vi "Arrange Panels.vi"(8 "error in":errorcluster, 11 "cPAS Facade in":refnum<class "cPAS Facade.lvclass">) -> (0 "error out":errorcluster, 3 "cPAS Facade out":refnum<class "cPAS Facade.lvclass">)   [LabVIEW 2015, in "cPAS Facade.lvclass"]
uses:
  cPAS Facade.lvclass
  UIs.ctl
  Reusable/GUI/Facade/GUI Facade.lvclass/GUI Facade.ctl
  Reusable/GUI/Facade/Accessors/Read sPanel.vi
  Reusable/GUI/Facade/Accessors/Read FP Refs.vi
  Reusable/GUI/Facade/Accessors/Write sPanel.vi
  Reusable/GUI/Facade/Accessors/Write FP Refs.vi
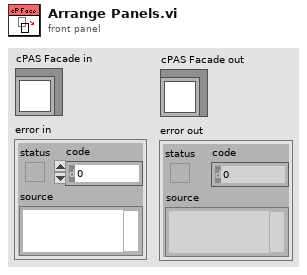
[diagram p1: front panel]
types:
  T1 = typedef "cPAS Facade.lvclass/UIs.ctl" = enum8{"PAS HF", "PAS Ctl", "PAS Der", "PAS HK", "Common", "Pcal", "CRD Ctl", "CRD RD", "CRD Der", "CRD HK", "Calibration", "CLAP", "Derived", "Housekeeping"}
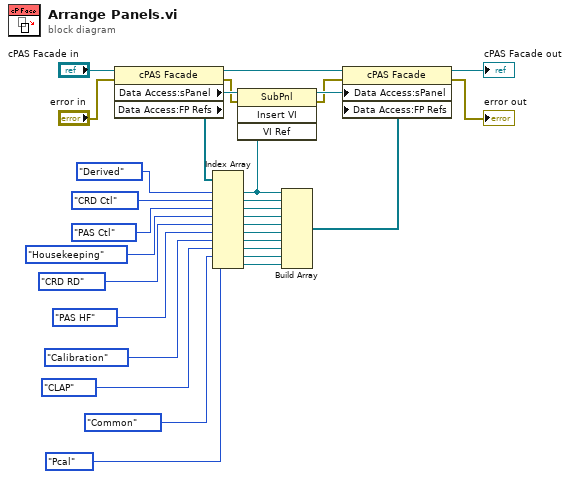
[diagram p0: block diagram]
diagram:
  n1 = property class="cPAS Facade"(reference="cPAS Facade in", error in="error in") -> (reference out=w23:refnum<class "cPAS Facade.lvclass">, error out=w2:errorcluster, "Data Access:sPanel"=w25:refnum<vi>, "Data Access:FP Refs"=w26:refnum<vi>[])
  n2 = Index Array(array=w26, index #1=UIs."Derived" ("UIs"), index #2=UIs."CRD Ctl" ("UIs"), index #3=UIs."PAS Ctl" ("UIs"), index #4=UIs."Housekeeping" ("UIs"), index #5=UIs."CRD RD" ("UIs"), index #6=UIs."PAS HF" ("UIs"), index #7=UIs."Calibration" ("UIs"), index #8=UIs."CLAP" ("UIs"), index #9=UIs."Common" ("UIs"), index #10=UIs."Pcal" ("UIs")) -> (element #1=w24:refnum<vi>, element #2=w30:refnum<vi>, element #3=w29:refnum<vi>, element #4=w28:refnum<vi>, element #5=w27:refnum<vi>, element #6=w11:refnum<vi>, element #7=w9:refnum<vi>, element #8=w7:refnum<vi>, element #9=w5:refnum<vi>, element #10=w3:refnum<vi>)
  n3 = invoke class="SubPnl" method="Insert VI"(reference=w25, error in=w2, "VI Ref"=w24) -> (reference out=w21:refnum<vi>, error out=w1:errorcluster)  [unwired: 1 in, 2 out]
  n4 = Build Array(w24, w30, w29, w28, w27, w11, w9, w7, w5, w3) -> (w22:refnum<vi>[])
  n5 = property class="cPAS Facade"(reference=w23, error in=w1, "Data Access:sPanel"=w21, "Data Access:FP Refs"=w22) -> (reference out=→"cPAS Facade out":refnum<class "cPAS Facade.lvclass">, error out=→"error out":errorcluster)
